vi "Station Initialize Guts.vi"(8 "error in (no error)":errorcluster, 11 "Station in":refnum<class "Station.lvclass">) -> (0 "error out":errorcluster, 2 "All Passed?":bool, 3 "Station out":refnum<class "Station.lvclass">)   [LabVIEW 2018, in "Station.lvclass"]
uses:
  Station.lvclass
  Station.lvclass/Station.ctl
  Controls/Server Control.ctl
  Generic Reuse/Logger/Log File Input.ctl
panel:
  out "Currently Initializing Instrument:":string
  # "Model Number:\nInstrument Number:\nRack ID:\nInst Mnemonic:\nComp Mnemonic:\nSubsys Mnemonic:\nIP Address:\nSub Address:\nFirmware Rev:\nExpected Options:\nRequired Options: \nExcluded Options:"
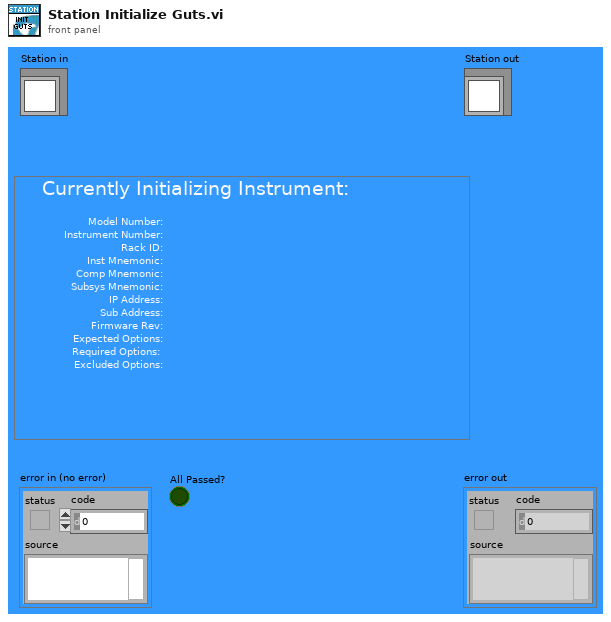
[diagram p1: front panel]
types:
  T1 = typedef "Server Control.ctl" = enum16{"Open New Reference", "Remove Reference", "Kill Server", "Set Station Ref", "Get Station Ref"}
  T2 = typedef "Log File Input.ctl" = cluster{"Log File Input":string, "Log Entry Type":enum16{"STANDARD", "WARNING", "CRITICAL"}}
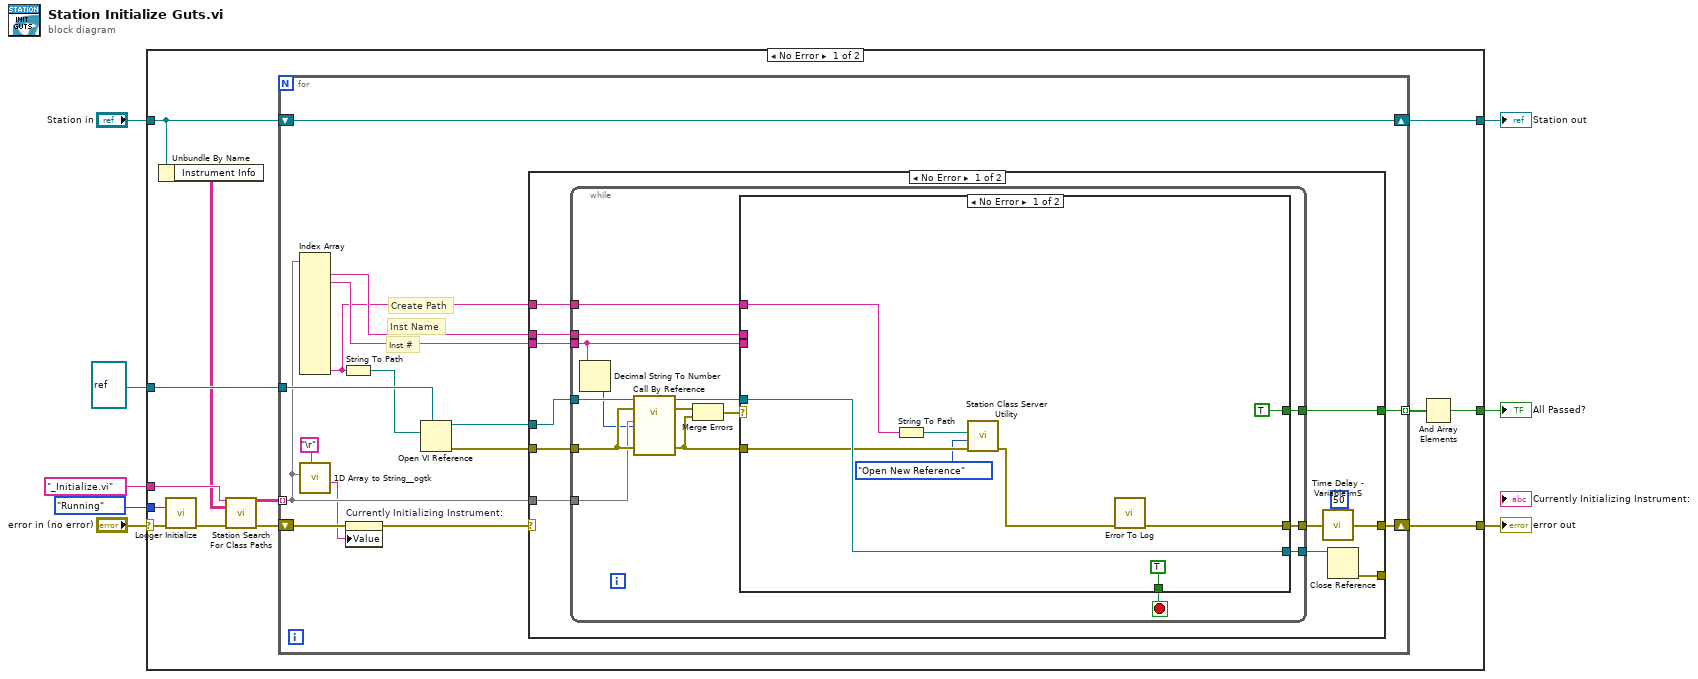
[diagram p0: block diagram]
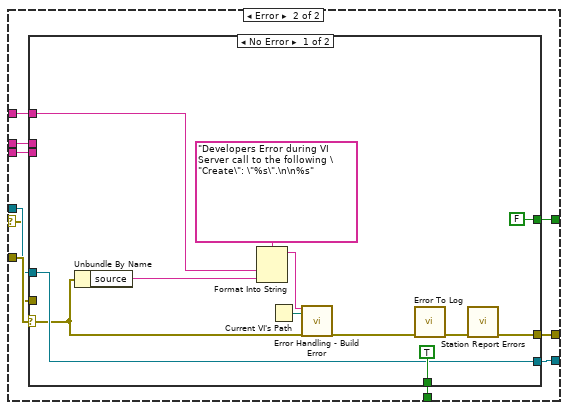
[diagram p2: hidden frame]
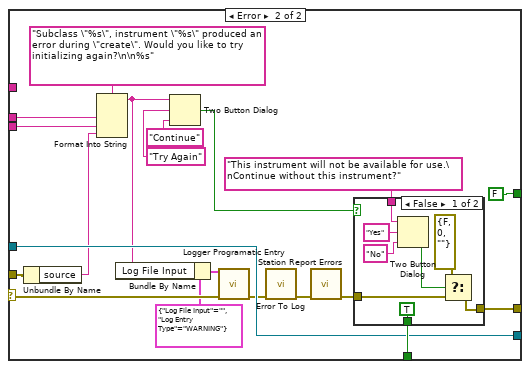
[diagram p3: hidden frame]
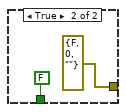
[diagram p4: hidden frame]
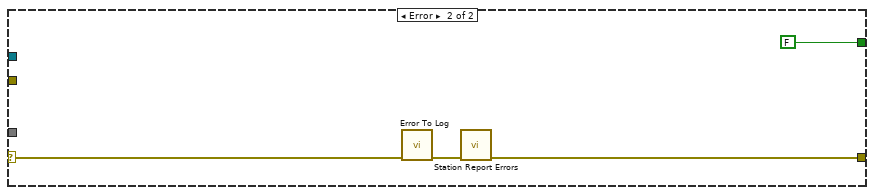
[diagram p5: hidden frame]
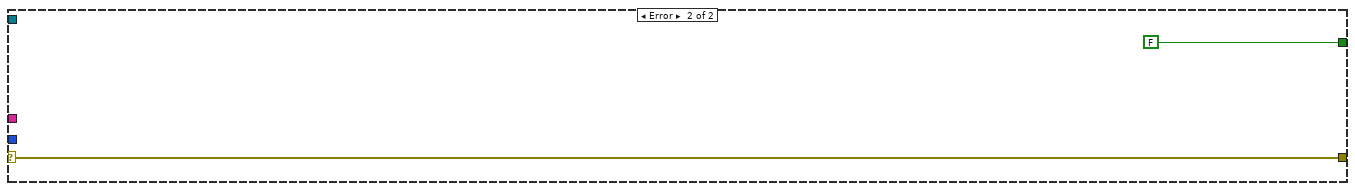
[diagram p6: hidden frame]
diagram:
  n1 = case shown="No Error" "error in (no error)" {
    selector: "error in (no error)" -> [w19 w130]
    tunnel: [w21 w130] -> w1
    tunnel: refnum<vi> refnum ("VI Refnum") -> [w17 _]
    tunnel: "_Initialize.vi" ("VI select") -> [w16 _]
    tunnel: enum16{"Running", "Closed"}."Running" ("Server Status") -> [w14 _]
    tunnel: [w12 FALSE] -> w5
    tunnel: "Station in" -> [w11 _]
    tunnel: [w9 _] -> w2
    frame No Error {
      n2 = Unbundle By Name(w11) -> ("Instrument Info"=w10:string[][])
      n3 = call "Logger Initialize.vi"("Server Status"=w14, "error in (no error)"=w19) -> ("error out"=w15:errorcluster)  [unwired: 13 in]
      n4 = call "Station Search For Class Paths.vi"("VI select"=w16, "Instrument Info"=w10, "error in (no error)"=w15) -> ("Updated Inst Info"=w18:string[][], "error out"=w20:errorcluster)  [unwired: 11 in]
      n5 = for {
        tunnel: w18 -> [w28] mode=indexing
        shift-right: [w30] -> w21
        shift-left: w20 -> [w25]
        tunnel: w17 -> [w36]
        tunnel: [w26] -> w13 mode=indexing
        shift-right: [w22] -> w9
        shift-left: w11 -> [w22]
        # "Inst #"
        # "Inst Name"
        # "Create Path"
        n6 = Index Array(array=w28) -> (element #1=w32:string, element #2=w31:string, element #13=w29:string)  [unwired: 13 in, 10 out]
        n7 = call <userlib>:"1D Array to String__ogtk.vi"("delimiter (Tab)"="\r", "Array of Strings"=w28) -> ("delimited string"=w23:string)  [unwired: 9 in]
        n8 = String To Path(string=w29) -> (path=w33:path)
        n9 = property on="Currently Initializing Instrument:" class="Str"(error in=w25, "Value"=w23) -> (error out=w24:errorcluster)  [unwired: 1 in, 1 out]
        n10 = Open VI Reference(type specifier VI Refnum (for type only)=w36, vi path=w33) -> (vi reference=w34:refnum<vi>, error out=w35:errorcluster)  [unwired: 4 in]
        n11 = case shown="No Error" w24 {
          selector: w24 -> [_ w128]
          tunnel: w35 -> [w47 _]
          tunnel: w34 -> [w48 _]
          tunnel: w32 -> [w46 _]
          tunnel: w31 -> [w45 _]
          tunnel: [w39 w126] -> w30
          tunnel: w29 -> [w44 _]
          tunnel: [w42 _] -> _
          tunnel: w28 -> [w41 _]
          tunnel: [w37 FALSE] -> w26
          frame No Error {
            n12 = while {
              tunnel: w48 -> [w63]
              tunnel: w47 -> [w62]
              tunnel: w46 -> [w61]
              tunnel: w45 -> [w50]
              tunnel: [w60] -> w40
              tunnel: w44 -> [w57]
              tunnel: [w53] -> w43
              tunnel: w41 -> [w52]
              tunnel: [w51] -> w37
              stop <- w56 stop-if-true
              n13 = Decimal String To Number(string=w50) -> (number=w49:i32)  [unwired: 2 in, 1 out]
              n14 = call-by-ref "?"(reference=w63, error in=w62, "Instrument Info"=w52, "User Reference"=w49, "error in (no error)"=w62) -> (reference out=w54:refnum<vi>, error out=w55:errorcluster, 19:"error out"=w58:errorcluster)  [unwired: 16 in]
              n15 = Merge Errors(w55, w58) -> (w59:errorcluster)
              n16 = case shown="No Error" w59 {
                selector: w59 -> [_ w74]
                tunnel: w58 -> [w69 w82]
                tunnel: w61 -> [_ w81]
                tunnel: w50 -> [_ w80]
                tunnel: [w66 w79] -> w60
                tunnel: w57 -> [w67 w78]
                tunnel: [TRUE w77] -> w56
                tunnel: w54 -> [w71 w76]
                tunnel: [w71 w75] -> w53
                tunnel: [TRUE w73] -> w51
                frame No Error {
                  n17 = String To Path(string=w67) -> (path=w68:path)
                  n18 = call "Station Class Server Utility.vi"("error in (no error)"=w69, "Action (0: Create)"=Server_Control."Open New Reference", "Creator Path (=\"\")"=w68) -> ("error out"=w70:errorcluster)  [unwired: 8 in]
                  n19 = call "Error To Log.vi"("error in (no error)"=w70) -> ("error out"=w66:errorcluster)  [unwired: 14 in]
                }
                frame Error {
                  n20 = case shown="No Error" w82 {
                    selector: w82 -> [w87 w103]
                    tunnel: w81 -> [_ w114]
                    tunnel: w80 -> [_ w112]
                    tunnel: [w84 w99] -> w79
                    tunnel: w78 -> [w90 _]
                    tunnel: [TRUE w107] -> w77
                    tunnel: w76 -> [w88 w106]
                    tunnel: [w88 w106] -> w75
                    tunnel: w74 -> [_ w105]
                    tunnel: [FALSE FALSE] -> w73
                    frame No Error {
                      n21 = Unbundle By Name(w87) -> ("source"=w86:string)
                      n22 = Format Into String(format string="Developers Error during VI Server call to the following \"Create\": \"%s\".\n\n%s", w90, w86) -> (resulting string=w92:string)  [unwired: 2 in, 1 out]
                      n23 = Current VI's Path() -> (path=w93:path)
                      n24 = call "Error Handling - Build Error.vi"("Error Message"=w92, "VI Path (calling VI path)"=w93, "error in (no error)"=w87) -> ("error out"=w94:errorcluster)  [unwired: 16 in]
                      n25 = call "Error To Log.vi"("error in (no error)"=w94) -> ("error out"=w85:errorcluster)  [unwired: 14 in]
                      n26 = call "Station Report Errors.vi"("error in (no error)"=w85) -> ("error out"=w84:errorcluster)  [unwired: 10 in]
                    }
                    frame Error {
                      n27 = Unbundle By Name(w105) -> ("source"=w104:string)
                      n28 = Format Into String(format string="Subclass \"%s\", instrument \"%s\" produced an error during \"create\". Would you like to try initializing again?\n\n%s", w114, w112, w104) -> (resulting string=w100:string)  [unwired: 2 in, 1 out]
                      n29 = Bundle By Name(cluster=T2 {"Log File Input"="", "Log Entry Type"=enum."WARNING"} ("Log File Input"), "Log File Input"=w100) -> (w102:T2)
                      n30 = Two Button Dialog(message=w100, 1:"Continue" ("F button name (\"Cancel\")"), 2:"Try Again" ("T button name (\"OK\")")) -> (T button?=w108:bool)
                      n31 = call "Logger Programatic Entry.vi"("Log File Input"=w102, "error in (no error)"=w103) -> ("error out"=w98:errorcluster)  [unwired: 13 in]
                      n32 = call "Error To Log.vi"("error in (no error)"=w98) -> ("error out"=w97:errorcluster)  [unwired: 14 in]
                      n33 = call "Station Report Errors.vi"("error in (no error)"=w97) -> ("error out"=w96:errorcluster)  [unwired: 10 in]
                      n34 = case shown="False" w108 {
                        tunnel: w96 -> [w122 _]
                        tunnel: [w120 errorcluster {"status"=FALSE, "code"=0, "source"=""}] -> w99
                        tunnel: "This instrument will not be available for use.\nContinue without this instrument?" -> [w116 _]
                        tunnel: [TRUE FALSE] -> w107
                        frame False {
                          n35 = Two Button Dialog(message=w116, 1:"No" ("F button name (\"Cancel\")"), 2:"Yes" ("T button name (\"OK\")")) -> (T button?=w119:bool)
                          n36 = Select(t=errorcluster {"status"=FALSE, "code"=0, "source"=""}, s=w119, f=w122) -> (s? t:f=w120:errorcluster)
                        }
                        frame True {
                        }
                      }
                    }
                  }
                }
              }
            }
            n37 = call "Time Delay - Variable mS.vi"("milliseconds to wait"=u32 50, "error in (no error)"=w40) -> ("error out"=w39:errorcluster)  [unwired: 2 in]
            n38 = Close Reference(reference=w43) -> (error out=w42:errorcluster)  [unwired: 1 in]
          }
          frame Error {
            n39 = call "Error To Log.vi"("error in (no error)"=w128) -> ("error out"=w127:errorcluster)  [unwired: 14 in]
            n40 = call "Station Report Errors.vi"("error in (no error)"=w127) -> ("error out"=w126:errorcluster)  [unwired: 10 in]
          }
        }
      }
      n41 = And Array Elements(Boolean array=w13) -> (logical AND=w12:bool)
    }
    frame Error {
    }
  }
  "error out" <- w1
  "Station out" <- w2
  "All Passed?" <- w5
